vi "Set Up Dialog - Heart Sounds.vi"() -> ()   [LabVIEW 2012]
panel:
  in  "SPN-304 Set Up":bool
  out "Calibration Instructions":string="1. Connect the sensor to your myDAQ as shown in the diagram above.\n\n2. Place the Spirometer (SPN-304) in the Heart Sounds (HS) mode, using the switch.\n\n3. Connect the Heart Sounds Sensor (HSMN-304) to the white connector of the Spirometer (SPN-304). \nOptionally, Plug the Red input of the SPN-304 using the RED blocking cap.\n."
  # "iWorx - Heart Sounds - Set Up"
  # "Heart Sounds Sensor (HSMN - 300)"
  # "iWorx"
  # "SPN-304"
  # "Sensor"
  # "myDAQ"
  # "Computer"
  # "HSMN - 300"
  # "(Spirometer)"
  # "Adaptor"
  # "Connection Diagram"
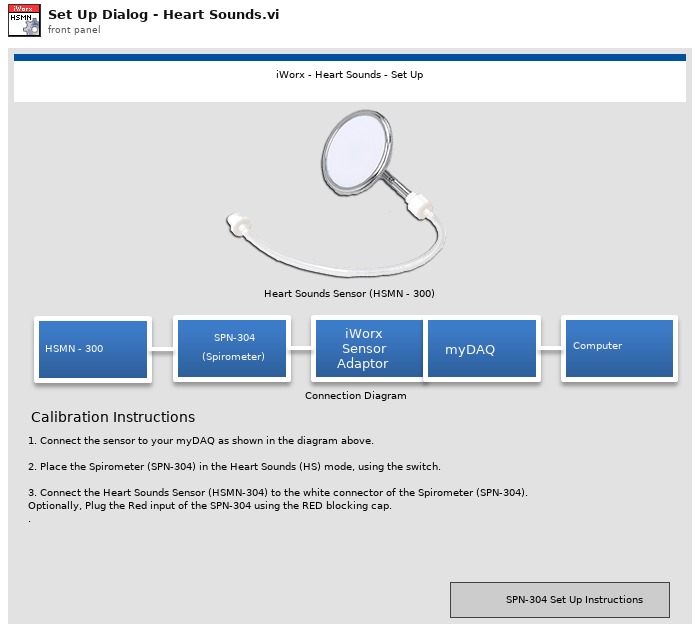
[diagram p1: front panel]
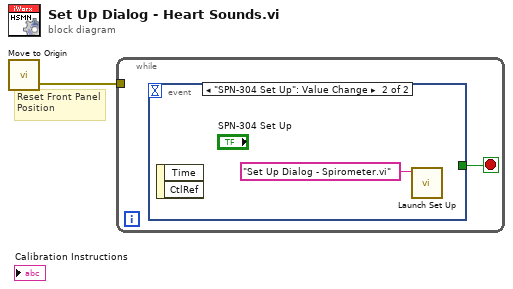
[diagram p0: block diagram]
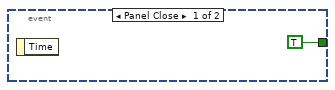
[diagram p2: hidden frame]
diagram:
  # "Reset Front Panel Position"
  n1 = call "Move to Origin.vi"() -> ("Error Out"=w1:errorcluster)  [unwired: 3 in]
  n2 = while {
    tunnel: w1 -> [_]
    stop <- w2 stop-if-true
    n3 = event shown="[1] \"SPN-304 Set Up\": Value Change" {
      selector: _ -> [_ _]
      dyn-events: _ -> [_ _]
      timeout: _ -> [_ _]
      tunnel: [TRUE _] -> w2
      event Panel Close {
        n4 = event-data() -> ()  [unwired: 1 in, 1 out]
      }
      event "SPN-304 Set Up": Value Change {
        n5 = event-data() -> ()  [unwired: 1 in, 2 out]
        n6 = call "Launch Set Up.vi"("name or relative path"="Set Up Dialog - Spirometer.vi") -> ()  [unwired: 9 in, 2 out]
      }
    }
  }
